vi "VNS Zobolas LSA Scheduler Selector.vi"(6 "Scheduler":T2, 7 "Objective":T1, 8 "error in (no error)":errorcluster, 9 "Reorder?":bool, 10 "Schedule in":u16[](array[numeric]), 11 "OSSP_Problem in":refnum<class "OSSP_Problem.lvclass">) -> (0 "error out":errorcluster, 1 "Total Tardiness (U16)":u16, 2 "Schedule out":u16[](array[numeric]), 3 "OSSP_Problem out":refnum<class "OSSP_Problem.lvclass">)   [LabVIEW 2013]
uses:
  GA/Controls/Scheduler Type.ctl
  Classes/OSSP_Problem.lvclass
  GA/Controls/Objective.ctl
  Classes/OSSP_Problem.lvclass/OSSP_Problem.ctl
  Classes/Scheduler_Class/Operation to Machine Job Tuple.vi
  Classes/Scheduler_Class/Prins FIFO Scheduler Methods and Controls/Prins FIFO Scheduler.vi
  Classes/Scheduler_Class/Prins FIFO Scheduler Methods and Controls/Methods/Calculate Final Completion Times of Jobs.vi
  Classes/Scheduler_Class/Prins FIFO Scheduler Methods and Controls/Methods/Reorder Schedule(Prins FIFO) based on Start Times.vi
  Classes/Scheduler_Class/Prins FIFO Scheduler Methods and Controls/Methods/UpdateMachineGaps.vi
  Classes/Scheduler_Class/Prins FIFO Scheduler Methods and Controls/Methods/UpdateJobGaps.vi
  Classes/Scheduler_Class/Prins FIFO Scheduler Methods and Controls/Methods/Find Intersecting Gaps.vi
  Classes/Scheduler_Class/GT Algorithm Find M_ok and J_ok.vi
  Classes/Scheduler_Class/Prins FIFO Scheduler Methods and Controls/Methods/Transform to Plain Job and Machine Gaps Array.vi
  Classes/Scheduler.lvclass
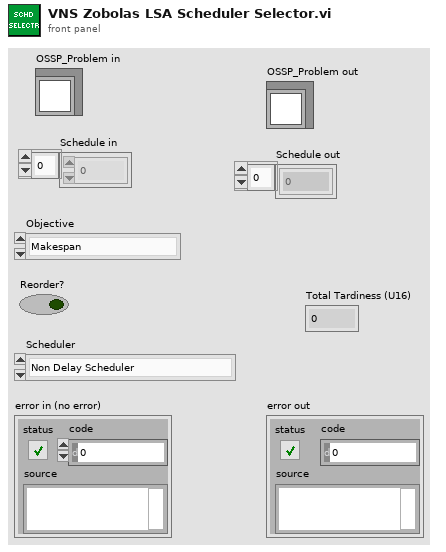
[diagram p1: front panel]
types:
  T1 = typedef "Objective.ctl" = enum16{"Makespan", "Total Tardiness"}
  T2 = typedef "Scheduler Type.ctl" = enum16{"Non Delay Scheduler", "GT Active Scheduler", "My Faulty Scheduler", "Prins FIFO Scheduler", "SemiActive Scheduler"}
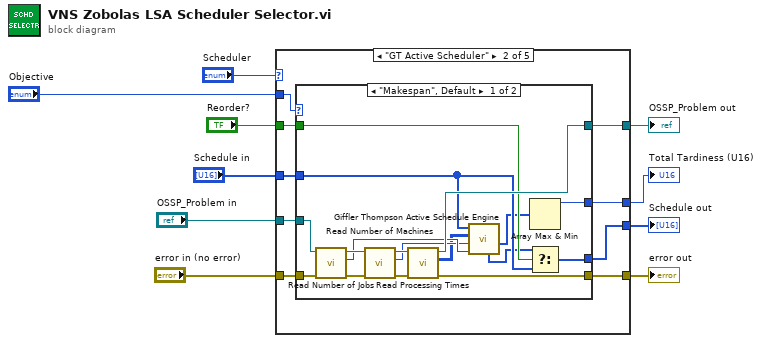
[diagram p0: block diagram]
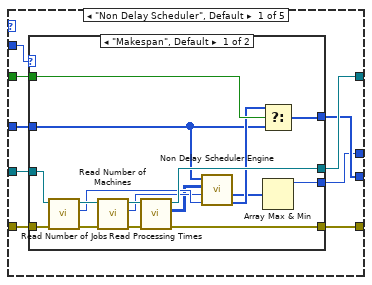
[diagram p2: hidden frame]
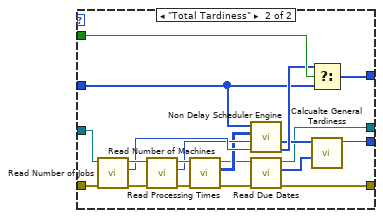
[diagram p3: hidden frame]
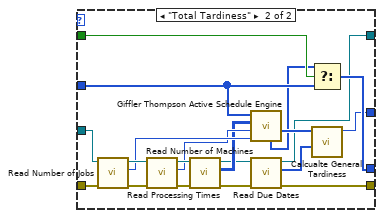
[diagram p4: hidden frame]
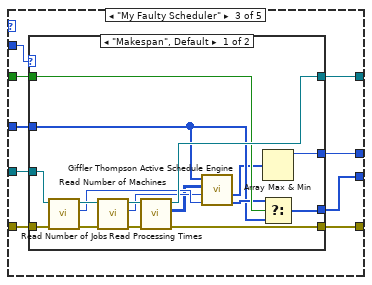
[diagram p5: hidden frame]
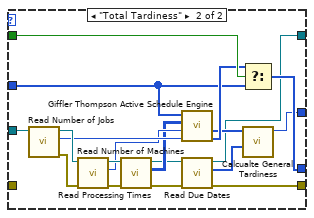
[diagram p6: hidden frame]
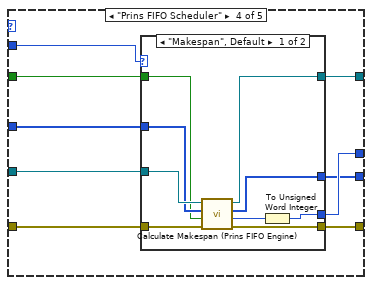
[diagram p7: hidden frame]
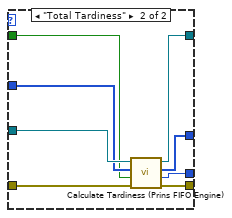
[diagram p8: hidden frame]
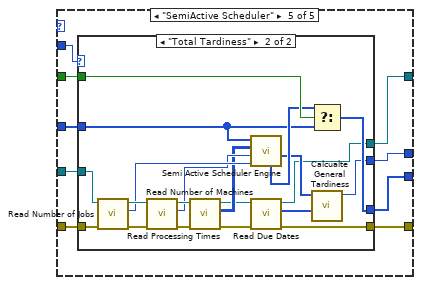
[diagram p9: hidden frame]
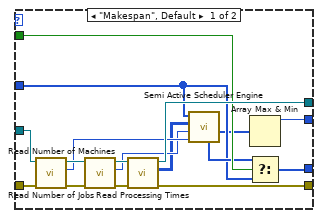
[diagram p10: hidden frame]
diagram:
  n1 = case shown="\"GT Active Scheduler\"" "Scheduler" {
    tunnel: [w11 w60 w104 w156 w175] -> w1
    tunnel: "Schedule in" -> [w14 w63 w110 w155 w181]
    tunnel: [w12 w59 w105 w154 w176] -> w3
    tunnel: "Objective" -> [w19 w57 w108 w153 w180]
    tunnel: "Reorder?" -> [w13 w62 w107 w152 w178]
    tunnel: [w17 w58 w103 w151 w174] -> w6
    tunnel: "OSSP_Problem in" -> [w18 w64 w111 w150 w182]
    tunnel: "error in (no error)" -> [w16 w65 w109 w149 w179]
    tunnel: [w15 w61 w106 w148 w177] -> w9
    frame "Non Delay Scheduler", Default {
      n2 = case shown="\"Makespan\", Default" w19 {
        tunnel: w18 -> [w36 w56]
        tunnel: [w33 w40] -> w17
        tunnel: w16 -> [w32 w53]
        tunnel: [w29 w39] -> w15
        tunnel: w14 -> [w23 w45]
        tunnel: w13 -> [w25 w47]
        tunnel: [w22 w44] -> w12
        tunnel: [w20 w37] -> w11
        frame "Makespan", Default {
          n3 = call "Read Number of Jobs.vi"("error in (no error)"=w32, "OSSP_Problem in"=w36) -> ("error out"=w31:errorcluster, "Number of Jobs"=w28:i32, "OSSP_Problem out"=w35:refnum<class "OSSP_Problem.lvclass">)  [unwired: 7 in]
          n4 = call "Read Number of Machines.vi"("error in (no error)"=w31, "OSSP_Problem in"=w35) -> ("error out"=w30:errorcluster, "Number of Machines"=w27:i32, "OSSP_Problem out"=w34:refnum<class "OSSP_Problem.lvclass">)  [unwired: 7 in]
          n5 = call "Read Processing Times.vi"("error in (no error)"=w30, "OSSP_Problem in"=w34) -> ("error out"=w29:errorcluster, "Processing Times"=w26:u16[][], "OSSP_Problem out"=w33:refnum<class "OSSP_Problem.lvclass">)  [unwired: 7 in]
          n6 = call "Non Delay Scheduler Engine.vi"("Number of  Jobs"=w28, "Number of Machines"=w27, "Processing Times"=w26, "Schedule"=w23) -> ("Reordered Schedule"=w24:u16[], "Job Completion Times"=w21:u16[])  [unwired: 2 in, 4 out]
          n7 = Select(t=w24, s=w25, f=w23) -> (s? t:f=w22:u16[])
          n8 = Array Max & Min(array=w21) -> (max value=w20:u16)  [unwired: 3 out]
        }
        frame "Total Tardiness" {
          n9 = call "Read Number of Jobs.vi"("error in (no error)"=w53, "OSSP_Problem in"=w56) -> ("error out"=w52:errorcluster, "Number of Jobs"=w50:i32, "OSSP_Problem out"=w55:refnum<class "OSSP_Problem.lvclass">)  [unwired: 7 in]
          n10 = call "Read Number of Machines.vi"("error in (no error)"=w52, "OSSP_Problem in"=w55) -> ("error out"=w51:errorcluster, "Number of Machines"=w49:i32, "OSSP_Problem out"=w54:refnum<class "OSSP_Problem.lvclass">)  [unwired: 7 in]
          n11 = call "Read Processing Times.vi"("error in (no error)"=w51, "OSSP_Problem in"=w54) -> ("error out"=w42:errorcluster, "Processing Times"=w48:u16[][], "OSSP_Problem out"=w41:refnum<class "OSSP_Problem.lvclass">)  [unwired: 7 in]
          n12 = call "Non Delay Scheduler Engine.vi"("Number of  Jobs"=w50, "Number of Machines"=w49, "Processing Times"=w48, "Schedule"=w45) -> ("Reordered Schedule"=w46:u16[], "Job Completion Times"=w43:u16[])  [unwired: 2 in, 4 out]
          n13 = call "Read Due Dates.vi"("error in (no error)"=w42, "OSSP_Problem in"=w41) -> ("error out"=w39:errorcluster, "Due Dates"=w38:u16[], "OSSP_Problem out"=w40:refnum<class "OSSP_Problem.lvclass">)  [unwired: 7 in]
          n14 = Select(t=w46, s=w47, f=w45) -> (s? t:f=w44:u16[])
          n15 = call "Calcualte General Tardiness.vi"("Due Dates"=w38, "Job Completion Times"=w43) -> ("Total Tardiness (U16)"=w37:u16)  [unwired: 9 in]
        }
      }
    }
    frame "GT Active Scheduler" {
      n16 = case shown="\"Makespan\", Default" w57 {
        tunnel: w64 -> [w82 w102]
        tunnel: [w79 w87] -> w58
        tunnel: w65 -> [w78 w99]
        tunnel: [w75 w86] -> w61
        tunnel: w63 -> [w70 w92]
        tunnel: w62 -> [w71 w93]
        tunnel: [w69 w91] -> w59
        tunnel: [w67 w84] -> w60
        frame "Makespan", Default {
          n17 = call "Read Number of Jobs.vi"("error in (no error)"=w78, "OSSP_Problem in"=w82) -> ("error out"=w77:errorcluster, "Number of Jobs"=w74:i32, "OSSP_Problem out"=w81:refnum<class "OSSP_Problem.lvclass">)  [unwired: 7 in]
          n18 = call "Read Number of Machines.vi"("error in (no error)"=w77, "OSSP_Problem in"=w81) -> ("error out"=w76:errorcluster, "Number of Machines"=w73:i32, "OSSP_Problem out"=w80:refnum<class "OSSP_Problem.lvclass">)  [unwired: 7 in]
          n19 = call "Read Processing Times.vi"("error in (no error)"=w76, "OSSP_Problem in"=w80) -> ("error out"=w75:errorcluster, "Processing Times"=w72:u16[][], "OSSP_Problem out"=w79:refnum<class "OSSP_Problem.lvclass">)  [unwired: 7 in]
          n20 = call "Giffler Thompson Active Schedule Engine.vi"("Number of  Jobs"=w74, "Number of Machines"=w73, "Processing Times"=w72, "Schedule In"=w70) -> ("Job Completion Times"=w68:u16[], "Ordered Schedule Out"=w66:u16[])  [unwired: 3 in, 3 out]
          n21 = Array Max & Min(array=w68) -> (max value=w67:u16)  [unwired: 3 out]
          n22 = Select(t=w66, s=w71, f=w70) -> (s? t:f=w69:u16[])
        }
        frame "Total Tardiness" {
          n23 = call "Read Number of Jobs.vi"("error in (no error)"=w99, "OSSP_Problem in"=w102) -> ("error out"=w98:errorcluster, "Number of Jobs"=w96:i32, "OSSP_Problem out"=w101:refnum<class "OSSP_Problem.lvclass">)  [unwired: 7 in]
          n24 = call "Read Number of Machines.vi"("error in (no error)"=w98, "OSSP_Problem in"=w101) -> ("error out"=w97:errorcluster, "Number of Machines"=w95:i32, "OSSP_Problem out"=w100:refnum<class "OSSP_Problem.lvclass">)  [unwired: 7 in]
          n25 = call "Read Processing Times.vi"("error in (no error)"=w97, "OSSP_Problem in"=w100) -> ("error out"=w89:errorcluster, "Processing Times"=w94:u16[][], "OSSP_Problem out"=w88:refnum<class "OSSP_Problem.lvclass">)  [unwired: 7 in]
          n26 = call "Giffler Thompson Active Schedule Engine.vi"("Number of  Jobs"=w96, "Number of Machines"=w95, "Processing Times"=w94, "Schedule In"=w92) -> ("Job Completion Times"=w90:u16[], "Ordered Schedule Out"=w83:u16[])  [unwired: 3 in, 3 out]
          n27 = call "Read Due Dates.vi"("error in (no error)"=w89, "OSSP_Problem in"=w88) -> ("error out"=w86:errorcluster, "Due Dates"=w85:u16[], "OSSP_Problem out"=w87:refnum<class "OSSP_Problem.lvclass">)  [unwired: 7 in]
          n28 = Select(t=w83, s=w93, f=w92) -> (s? t:f=w91:u16[])
          n29 = call "Calcualte General Tardiness.vi"("Due Dates"=w85, "Job Completion Times"=w90) -> ("Total Tardiness (U16)"=w84:u16)  [unwired: 9 in]
        }
      }
    }
    frame "My Faulty Scheduler" {
      n30 = case shown="\"Makespan\", Default" w108 {
        tunnel: w111 -> [w128 w147]
        tunnel: [w125 w132] -> w103
        tunnel: [w122 w131] -> w106
        tunnel: w110 -> [w116 w137]
        tunnel: w107 -> [w118 w139]
        tunnel: [w115 w136] -> w105
        tunnel: [w113 w129] -> w104
        tunnel: w109 -> [w112 _]
        frame "Makespan", Default {
          n31 = call "Read Number of Jobs.vi"("error in (no error)"=w112, "OSSP_Problem in"=w128) -> ("error out"=w124:errorcluster, "Number of Jobs"=w121:i32, "OSSP_Problem out"=w127:refnum<class "OSSP_Problem.lvclass">)  [unwired: 7 in]
          n32 = call "Read Number of Machines.vi"("error in (no error)"=w124, "OSSP_Problem in"=w127) -> ("error out"=w123:errorcluster, "Number of Machines"=w120:i32, "OSSP_Problem out"=w126:refnum<class "OSSP_Problem.lvclass">)  [unwired: 7 in]
          n33 = call "Read Processing Times.vi"("error in (no error)"=w123, "OSSP_Problem in"=w126) -> ("error out"=w122:errorcluster, "Processing Times"=w119:u16[][], "OSSP_Problem out"=w125:refnum<class "OSSP_Problem.lvclass">)  [unwired: 7 in]
          n34 = call "Giffler Thompson Active Schedule Engine.vi"("Number of  Jobs"=w121, "Number of Machines"=w120, "Processing Times"=w119, "Schedule In"=w116) -> ("Machine Completion Times"=w117:u16[], "Job Completion Times"=w114:u16[])  [unwired: 3 in, 3 out]
          n35 = Array Max & Min(array=w114) -> (max value=w113:u16)  [unwired: 3 out]
          n36 = Select(t=w117, s=w118, f=w116) -> (s? t:f=w115:u16[])
        }
        frame "Total Tardiness" {
          n37 = call "Read Number of Jobs.vi"("OSSP_Problem in"=w147) -> ("error out"=w144:errorcluster, "Number of Jobs"=w142:i32, "OSSP_Problem out"=w146:refnum<class "OSSP_Problem.lvclass">)  [unwired: 8 in]
          n38 = call "Read Number of Machines.vi"("error in (no error)"=w144, "OSSP_Problem in"=w146) -> ("error out"=w143:errorcluster, "Number of Machines"=w141:i32, "OSSP_Problem out"=w145:refnum<class "OSSP_Problem.lvclass">)  [unwired: 7 in]
          n39 = call "Read Processing Times.vi"("error in (no error)"=w143, "OSSP_Problem in"=w145) -> ("error out"=w134:errorcluster, "Processing Times"=w140:u16[][], "OSSP_Problem out"=w133:refnum<class "OSSP_Problem.lvclass">)  [unwired: 7 in]
          n40 = call "Giffler Thompson Active Schedule Engine.vi"("Number of  Jobs"=w142, "Number of Machines"=w141, "Processing Times"=w140, "Schedule In"=w137) -> ("Machine Completion Times"=w138:u16[], "Job Completion Times"=w135:u16[])  [unwired: 3 in, 3 out]
          n41 = call "Read Due Dates.vi"("error in (no error)"=w134, "OSSP_Problem in"=w133) -> ("error out"=w131:errorcluster, "Due Dates"=w130:u16[], "OSSP_Problem out"=w132:refnum<class "OSSP_Problem.lvclass">)  [unwired: 7 in]
          n42 = Select(t=w138, s=w139, f=w137) -> (s? t:f=w136:u16[])
          n43 = call "Calcualte General Tardiness.vi"("Due Dates"=w130, "Job Completion Times"=w135) -> ("Total Tardiness (U16)"=w129:u16)  [unwired: 9 in]
        }
      }
    }
    frame "Prins FIFO Scheduler" {
      n44 = case shown="\"Makespan\", Default" w153 {
        tunnel: [w164 w172] -> w156
        tunnel: w155 -> [w160 w169]
        tunnel: [w165 w173] -> w154
        tunnel: w152 -> [w159 w168]
        tunnel: w150 -> [w161 w171]
        tunnel: [w158 w170] -> w151
        tunnel: w149 -> [w162 w167]
        tunnel: [w157 w166] -> w148
        frame "Makespan", Default {
          n45 = call "Calculate Makespan (Prins FIFO Engine).vi"("error in (no error)"=w162, "Reorder?"=w159, "Schedule In"=w160, "OSSP_Problem in"=w161) -> ("error out"=w157:errorcluster, "Makespan"=w163:i32, "Schedule Out"=w165:u16[], "OSSP_Problem out"=w158:refnum<class "OSSP_Problem.lvclass">)  [unwired: 4 in]
          n46 = To Unsigned Word Integer(number=w163) -> (unsigned 16bit integer=w164:u16)
        }
        frame "Total Tardiness" {
          n47 = call "Calculate Tardiness (Prins FIFO Engine).vi"("error in (no error)"=w167, "Reorder?"=w168, "Schedule In"=w169, "OSSP_Problem in"=w171) -> ("error out"=w166:errorcluster, "Tardiness(Prins FIFO Engine)"=w172:u16, "Schedule Out"=w173:u16[], "OSSP_Problem out"=w170:refnum<class "OSSP_Problem.lvclass">)  [unwired: 3 in, 1 out]
        }
      }
    }
    frame "SemiActive Scheduler" {
      n48 = case shown="\"Total Tardiness\"" w180 {
        tunnel: w182 -> [w199 w219]
        tunnel: [w196 w203] -> w174
        tunnel: w179 -> [w195 w216]
        tunnel: [w192 w202] -> w177
        tunnel: w181 -> [w186 w208]
        tunnel: w178 -> [w188 w210]
        tunnel: [w185 w207] -> w176
        tunnel: [w183 w200] -> w175
        frame "Makespan", Default {
          n49 = call "Read Number of Jobs.vi"("error in (no error)"=w195, "OSSP_Problem in"=w199) -> ("error out"=w194:errorcluster, "Number of Jobs"=w191:i32, "OSSP_Problem out"=w198:refnum<class "OSSP_Problem.lvclass">)  [unwired: 7 in]
          n50 = call "Read Number of Machines.vi"("error in (no error)"=w194, "OSSP_Problem in"=w198) -> ("error out"=w193:errorcluster, "Number of Machines"=w190:i32, "OSSP_Problem out"=w197:refnum<class "OSSP_Problem.lvclass">)  [unwired: 7 in]
          n51 = call "Read Processing Times.vi"("error in (no error)"=w193, "OSSP_Problem in"=w197) -> ("error out"=w192:errorcluster, "Processing Times"=w189:u16[][], "OSSP_Problem out"=w196:refnum<class "OSSP_Problem.lvclass">)  [unwired: 7 in]
          n52 = call "Semi Active Scheduler Engine.vi"("Number of  Jobs"=w191, "Number of Machines"=w190, "Processing Times"=w189, "Schedule"=w186) -> ("Job Completion Times"=w184:u16[], "Machine Completion Times"=w187:u16[])  [unwired: 3 in, 3 out]
          n53 = Array Max & Min(array=w184) -> (max value=w183:u16)  [unwired: 3 out]
          n54 = Select(t=w187, s=w188, f=w186) -> (s? t:f=w185:u16[])
        }
        frame "Total Tardiness" {
          n55 = call "Read Number of Jobs.vi"("error in (no error)"=w216, "OSSP_Problem in"=w219) -> ("error out"=w215:errorcluster, "Number of Jobs"=w213:i32, "OSSP_Problem out"=w218:refnum<class "OSSP_Problem.lvclass">)  [unwired: 7 in]
          n56 = call "Read Number of Machines.vi"("error in (no error)"=w215, "OSSP_Problem in"=w218) -> ("error out"=w214:errorcluster, "Number of Machines"=w212:i32, "OSSP_Problem out"=w217:refnum<class "OSSP_Problem.lvclass">)  [unwired: 7 in]
          n57 = call "Read Processing Times.vi"("error in (no error)"=w214, "OSSP_Problem in"=w217) -> ("error out"=w205:errorcluster, "Processing Times"=w211:u16[][], "OSSP_Problem out"=w204:refnum<class "OSSP_Problem.lvclass">)  [unwired: 7 in]
          n58 = call "Semi Active Scheduler Engine.vi"("Number of  Jobs"=w213, "Number of Machines"=w212, "Processing Times"=w211, "Schedule"=w208) -> ("Job Completion Times"=w206:u16[], "Machine Completion Times"=w209:u16[])  [unwired: 3 in, 3 out]
          n59 = call "Read Due Dates.vi"("error in (no error)"=w205, "OSSP_Problem in"=w204) -> ("error out"=w202:errorcluster, "Due Dates"=w201:u16[], "OSSP_Problem out"=w203:refnum<class "OSSP_Problem.lvclass">)  [unwired: 7 in]
          n60 = Select(t=w209, s=w210, f=w208) -> (s? t:f=w207:u16[])
          n61 = call "Calcualte General Tardiness.vi"("Due Dates"=w201, "Job Completion Times"=w206) -> ("Total Tardiness (U16)"=w200:u16)  [unwired: 9 in]
        }
      }
    }
  }
  "error out" <- w9
  "OSSP_Problem out" <- w6
  "Schedule out" <- w3
  "Total Tardiness (U16)" <- w1
